vi "TestIVLoader.vi"() -> ()   [LabVIEW 2020]
uses:
  <vilib>/Utility/file.llb/Read Delimited Spreadsheet (DBL).vi
panel:
  out "XY Graph":cluster{"all rows":dbl[], "all rows":dbl[]}(graph)
  out "all rows":dbl[][](array[numeric])
  in  "Path":path
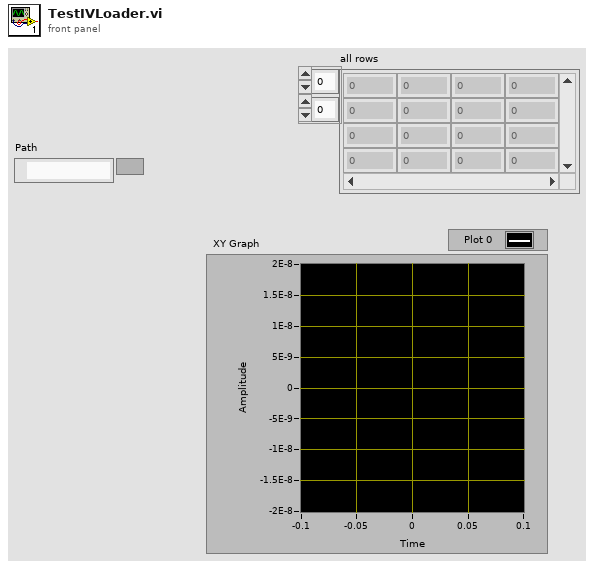
[diagram p1: front panel]
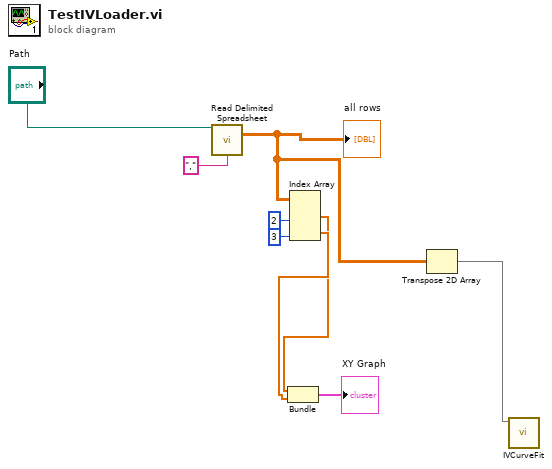
[diagram p0: block diagram]
diagram:
  n1 = call-poly <vilib>:"Read Delimited Spreadsheet.vi"("file path (dialog if empty)"="Path", "delimiter (\\t)"="," ("delimiter (\\t)")) -> ("all rows"=w2:dbl[][])  [unwired: 8 in, 5 out]
  "all rows" <- w2
  n2 = Index Array(array=w2, index (col) #1=2 ("disabled index (col)"), index (col) #2=3 ("index (col)")) -> (element #1=w3:dbl[], element #2=w4:dbl[])  [unwired: 2 in]
  n3 = Bundle("all rows"=w3, "all rows"=w4) -> (→"XY Graph":cluster{"all rows":dbl[], "all rows":dbl[]})  [unwired: 1 in]
  n4 = Transpose 2D Array(2D array=w2) -> (transposed array=w1:dbl[][])
  n5 = call "IVCurveFit.vi"("IVData"=w1) -> ()  [unwired: 7 in, 4 out]
